vi "TWM Measure.vi"(4 "TWM Status ref":refnum<vi>, 6 "TWM pipe":string, 8 "error in (no error)":errorcluster, 10 "TWM Measurement properties":T1={"Sampling frequency (Hz)"=500000.0, "Record length (multiples of period)"=1000.0, "Signal amplitude (V)"=4.5, "Measurement frequency (Hz)"=1000.0, "Calculate RMS from samples"=FALSE, "Algorithm"="TWM-WFFT", "Measurement path"=""} {"Measurement frequency (Hz)" format="%#_3p"; "Record length (multiples of period)" format="%#_3p"; "Sampling frequency (Hz)" format="%#_3p"}, 11 "TWM handle":i32) -> (0 "error out":errorcluster, 2 "TWM result as string":string[][](array[string]), 3 "TWM handle out":i32)   [LabVIEW 2020]
doc: "Set TWM measurement, initiate TWM measurement, wait for results if needed, reset connection if error."
uses:
  Type definitions/Sampling properties.ctl
  external libraries/TWM-1.8.7.0-client/TWM Client Quantity Record.ctl
  external libraries/TWM-1.8.7.0-client/TWM Client.lvlib
  external libraries/varilib/varilib.lvlib
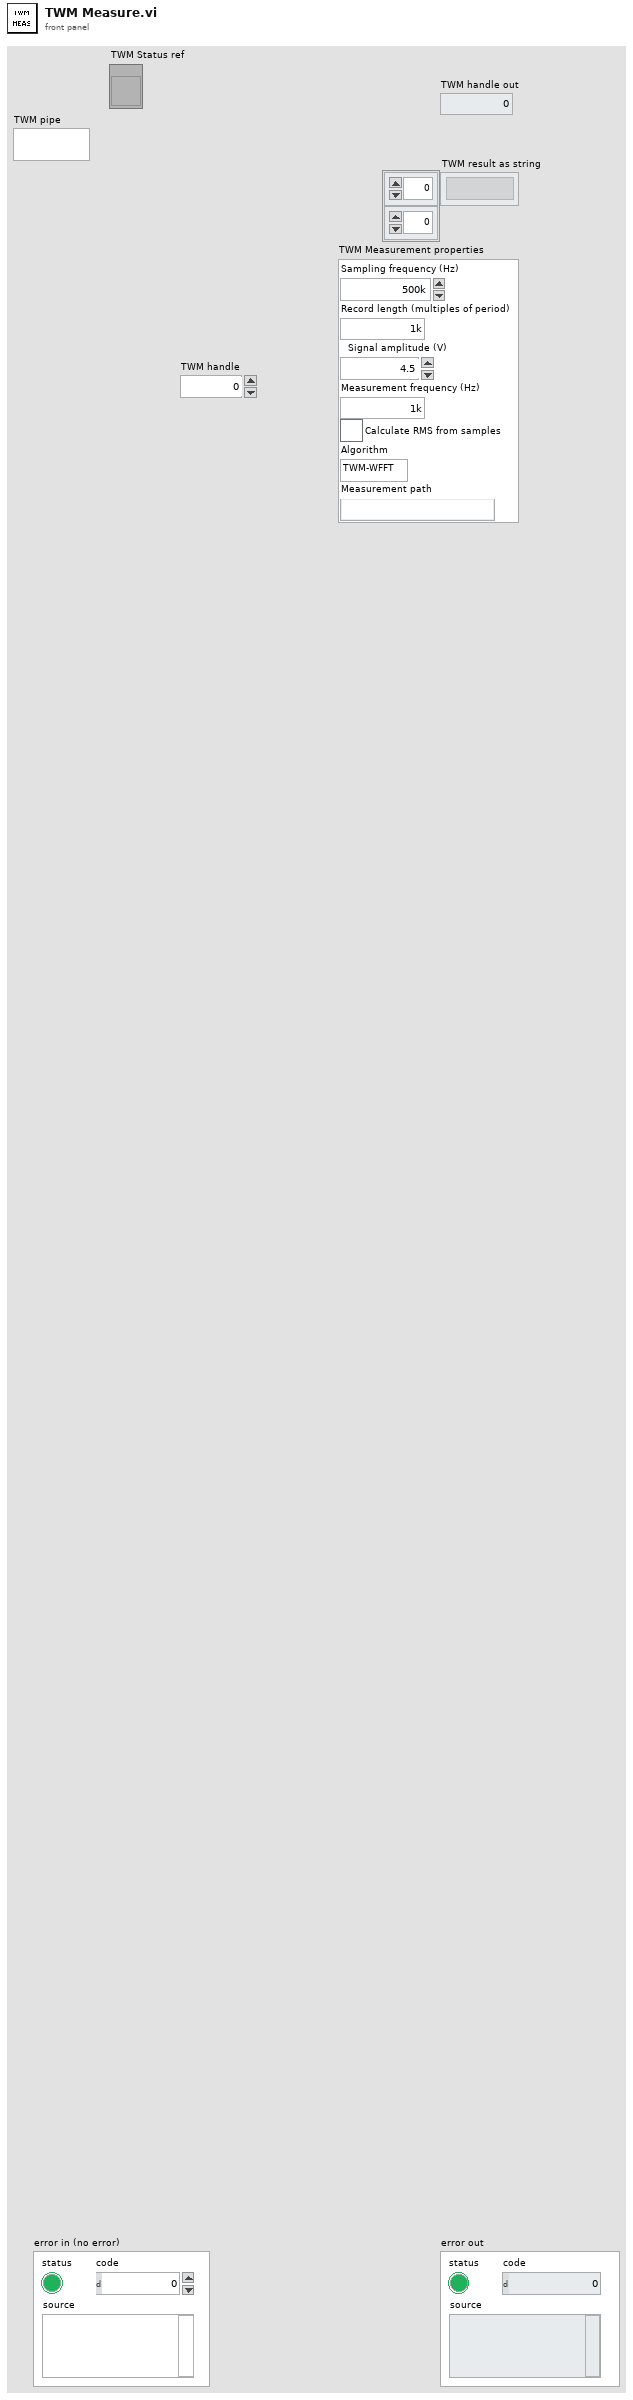
[diagram p1: front panel]
types:
  T1 = typedef "Sampling properties.ctl" = cluster{"Sampling frequency (Hz)":dbl, "Record length (multiples of period)":dbl, "Signal amplitude (V)":dbl, "Measurement frequency (Hz)":dbl, "Calculate RMS from samples":bool, "Algorithm":string, "Measurement path":string}
  T2 = typedef "TWM Client.lvlib/TWM Client Quantity Record.ctl" = cluster{"val":dbl[], "unc":dbl[], "name":string, "is valid?":bool, "has unc?":bool, "numel":i32, "ua":dbl[], "is phase?":bool, "is amplitude?":bool, "description":string, "phase tag":string, "num format":string, "is string?":bool, "string value":string}
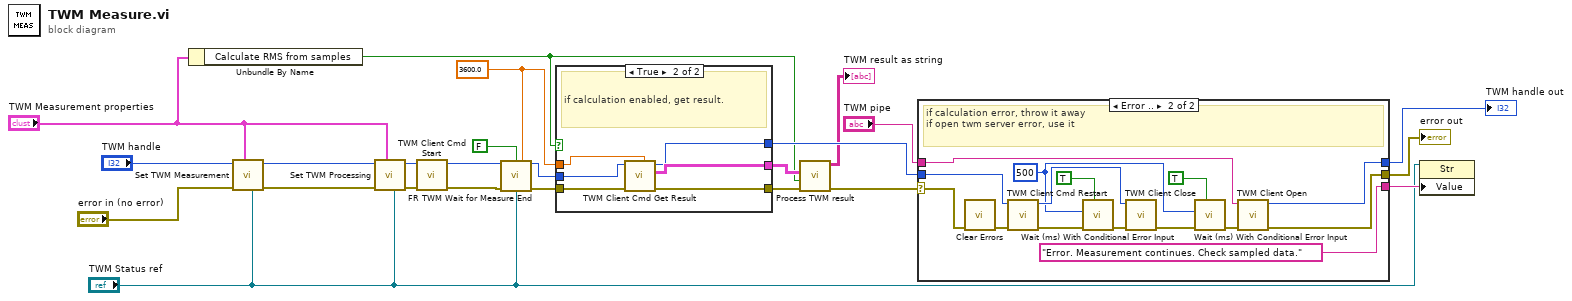
[diagram p0: block diagram]
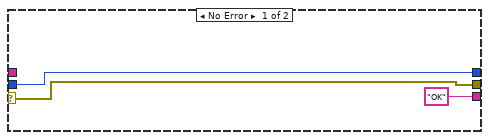
[diagram p2: hidden frame]
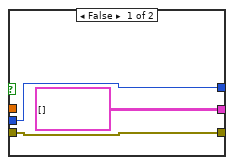
[diagram p3: hidden frame]
diagram:
  w21 = 3600.0 ("timeout [s] (10s)")
  n1 = Unbundle By Name("TWM Measurement properties") -> ("Calculate RMS from samples"=w4:bool)
  n2 = call "Set TWM Measurement.vi"("status ref (none)"="TWM Status ref", "TWM Measurement properties"="TWM Measurement properties", "error in"="error in (no error)", "TWM handle"="TWM handle") -> ("error out"=w9:errorcluster, "TWM handle out"=w12:i32)  [unwired: 6 in]
  n3 = call "Set TWM Processing.vi"("status ref (none)"="TWM Status ref", "TWM Measurement properties"="TWM Measurement properties", "error in"=w9, "handle"=w12) -> ("error out"=w10:errorcluster, "handle out"=w11:i32)  [unwired: 6 in]
  n4 = call "TWM Client Cmd Start.vi"("error in"=w10, "handle"=w11) -> ("error out"=w5:errorcluster, "handle out"=w6:i32)  [unwired: 8 in]
  n5 = call "FR TWM Wait for Measure End.vi"("handle"=w6, "Obtain results? (False)"=FALSE, "timeout [s] (10s)"=w21, "error in"=w5, "status ref (none)"="TWM Status ref") -> ("handle out"=w18:i32, "error out"=w17:errorcluster)  [unwired: 6 in, 3 out]
  n6 = case shown="True" w4 {
    tunnel: [T2[][] [] ("result data") w33] -> w14
    tunnel: w18 -> [w26 w32]
    tunnel: w17 -> [w25 w31]
    tunnel: [w26 w30] -> w19
    tunnel: w21 -> [_ w29]
    tunnel: [w25 w28] -> w22
    frame False {
    }
    frame True {
      # "if calculation enabled, get result."
      n7 = call "TWM Client Cmd Get Result.vi"("timeout [s] (10s)"=w29, "error in"=w31, "handle"=w32) -> ("error out"=w28:errorcluster, "result data"=w33:T2[][], "handle out"=w30:i32)  [unwired: 5 in, 1 out]
    }
  }
  n8 = call "Process TWM result.vi"("error from TWM get result"=w22, "Calculate RMS from samples"=w4, "TWM result"=w14) -> ("error out"=w23:errorcluster, "TWM result as string"=→"TWM result as string":string[][])  [unwired: 7 in]
  n9 = case shown="Error .." w23 {
    selector: w23 -> [w36 w51]
    tunnel: [w36 w47] -> w16
    tunnel: w19 -> [w35 w50]
    tunnel: [w35 w46] -> w20
    tunnel: ["OK" ("Value") "Error. Measurement continues. Check sampled data." ("Value")] -> w24
    tunnel: "TWM pipe" -> [_ w37]
    frame No Error {
    }
    frame Error {
      w39 = u32 500 ("milliseconds to wait")
      # "if calculation error, throw it away\nif open twm server error, use it"
      n10 = call <vilib>:"Clear Errors.vi"("error in (no error)"=w51) -> ("error out"=w49:errorcluster)  [unwired: 5 in, 1 out]
      n11 = call "TWM Client Cmd Restart.vi"("error in"=w49, "handle"=w50) -> ("error out"=w45:errorcluster, "handle out"=w48:i32)  [unwired: 8 in]
      n12 = call "Wait (ms) With Conditional Error Input.vi"("wait if error (F)"=TRUE, "error in (no error)"=w45, "milliseconds to wait"=w39) -> ("error out"=w44:errorcluster)  [unwired: 7 in, 1 out]
      n13 = call "TWM Client Close.vi"("error in"=w44, "handle in"=w48) -> ("error out"=w43:errorcluster)  [unwired: 9 in]
      n14 = call "Wait (ms) With Conditional Error Input.vi"("wait if error (F)"=TRUE, "error in (no error)"=w43, "milliseconds to wait"=w39) -> ("error out"=w42:errorcluster)  [unwired: 7 in, 1 out]
      n15 = call "TWM Client Open.vi"("error in"=w42, "pipe name"=w37) -> ("error out"=w47:errorcluster, "handle out"=w46:i32)  [unwired: 8 in]
    }
  }
  "TWM handle out" <- w20
  "error out" <- w16
  n16 = property class="Str"(reference="TWM Status ref", "Value"=w24) -> ()  [unwired: 1 in, 2 out]
